vi "loop timing.vi"() -> ()   [LabVIEW 2013]
uses:
  <vilib>/DAQmx/read.llb/DAQmx Read (Digital Bool 1Line 1Point).vi
  <vilib>/DAQmx/write.llb/DAQmx Write (Digital Bool 1Line 1Point).vi
  <vilib>/DAQmx/create/channels.llb/DAQmx Create Channel (DI-Digital Input).vi
  <vilib>/DAQmx/create/channels.llb/DAQmx Create Channel (DO-Digital Output).vi
  <vilib>/DAQmx/miscellaneous.llb/DAQmx Fill In Error Info.vi
panel:
  out "error out 2":errorcluster
  out "error out":errorcluster
  in  "DAQmx DO":tag="Dev1/port0/line1"
  in  "DAQmx DI":tag="Dev1/port0/line0"
  out "Max":dbl=8.0 format="%_6g"
  in  "stop":bool
  out "Average":dbl=1.0015833898416784 format="%_6g"
  out "Delay":dbl=1.0 format="%_6g"
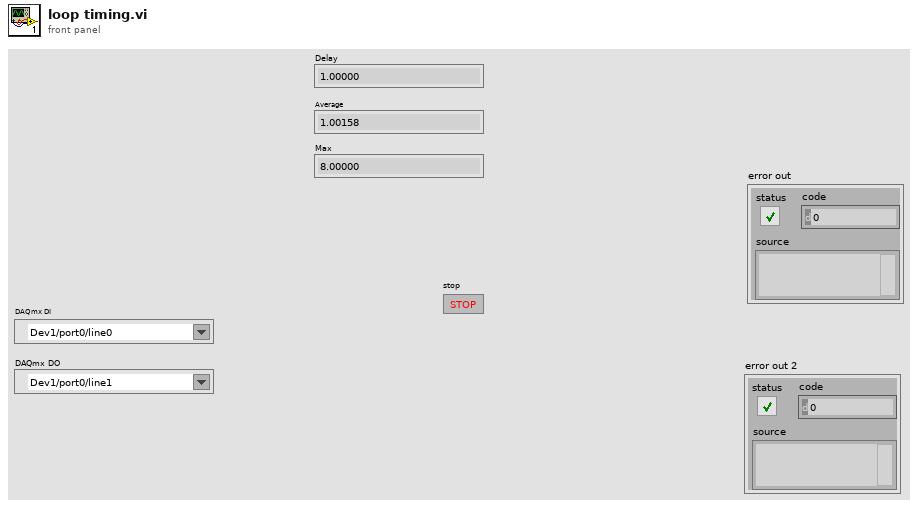
[diagram p1: front panel]
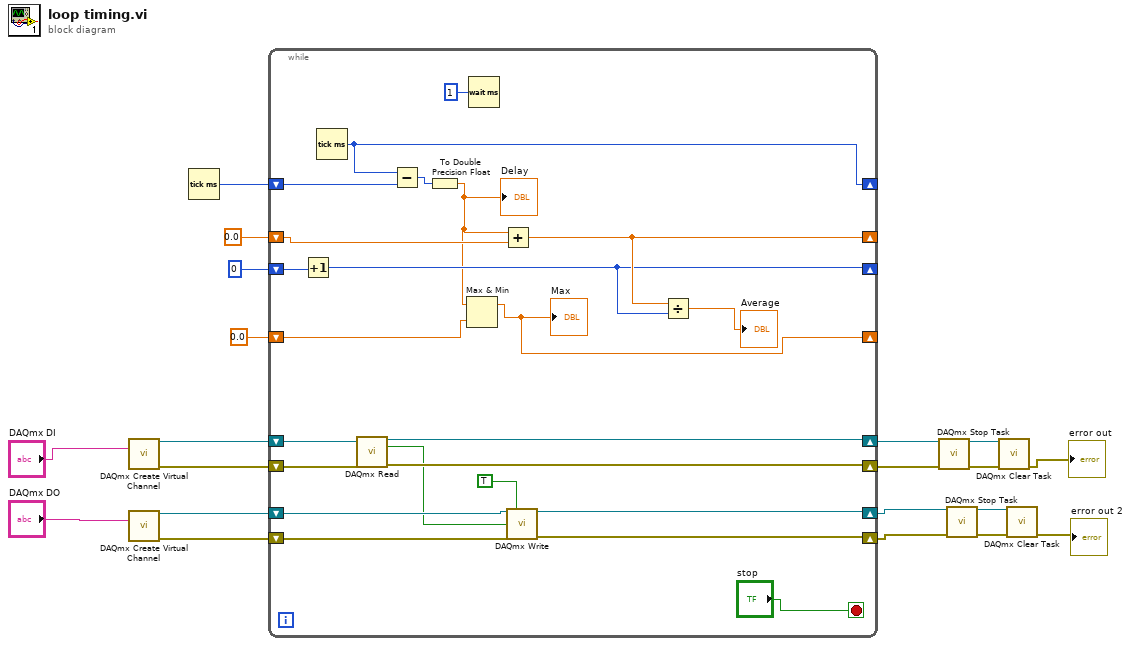
[diagram p0: block diagram]
diagram:
  n1 = call-poly <vilib>:"DAQmx Create Virtual Channel.vi"("lines"="DAQmx DI") -> ("task out"=w14:refnum<k21>, "error out"=w11:errorcluster)  [unwired: 13 in]
  n2 = call-poly <vilib>:"DAQmx Create Virtual Channel.vi"("lines"="DAQmx DO") -> ("task out"=w13:refnum<k21>, "error out"=w12:errorcluster)  [unwired: 13 in]
  n3 = Tick Count (ms)() -> (millisecond timer value=w20:u32)
  n4 = while {
    shift-right: [w40] -> _
    shift-left: w20 -> [w41]
    shift-right: [w36] -> _
    shift-left: 0.0 -> [w38]
    shift-right: [w35] -> _
    shift-left: 0 -> [w39]
    shift-right: [w31] -> _
    shift-left: 0.0 -> [w33]
    shift-right: [w29] -> w6
    shift-left: w13 -> [w30]
    shift-right: [w24] -> w4
    shift-left: w14 -> [w26]
    shift-right: [w27] -> w5
    shift-left: w12 -> [w28]
    shift-right: [w23] -> w3
    shift-left: w11 -> [w25]
    stop <- "stop" stop-if-true
    n5 = Increment(x=w39) -> (x+1=w35:i32)
    n6 = Tick Count (ms)() -> (millisecond timer value=w40:u32)
    n7 = call-poly <vilib>:"DAQmx Read.vi"("task/channels in"=w26, "error in"=w25) -> ("task out"=w24:refnum<k21>, "data"=w21:bool, "error out"=w23:errorcluster)  [unwired: 11 in]
    n8 = Subtract(x=w40, y=w41) -> (x-y=w37:u32)
    n9 = To Double Precision Float(number=w37) -> (double precision float=w32:dbl)
    "Delay" <- w32
    n10 = Max & Min(x=w32, y=w33) -> (max(x,y)=w31:dbl)  [unwired: 1 out]
    "Max" <- w31
    n11 = Wait (ms)(milliseconds to wait=u32 1) -> ()  [unwired: 1 out]
    n12 = Add(x=w32, y=w38) -> (x+y=w36:dbl)
    n13 = call-poly <vilib>:"DAQmx Write.vi"("task/channels in"=w30, "auto start"=TRUE, "data"=w21, "error in"=w28) -> ("task out"=w29:refnum<k21>, "error out"=w27:errorcluster)  [unwired: 9 in, 1 out]
    n14 = Divide(x=w36, y=w35) -> (x/y=→"Average":dbl)
  }
  n15 = call <vilib>:"DAQmx Stop Task.vi"("task/channels in"=w4, "error in"=w3) -> ("task out"=w10:refnum<k21>, "error out"=w9:errorcluster)  [unwired: 12 in]
  n16 = call <vilib>:"DAQmx Stop Task.vi"("task/channels in"=w6, "error in"=w5) -> ("task out"=w8:refnum<k21>, "error out"=w7:errorcluster)  [unwired: 12 in]
  n17 = call <vilib>:"DAQmx Clear Task.vi"("task in"=w10, "error in"=w9) -> ("error out"=→"error out":errorcluster)  [unwired: 13 in]
  n18 = call <vilib>:"DAQmx Clear Task.vi"("task in"=w8, "error in"=w7) -> ("error out"=→"error out 2":errorcluster)  [unwired: 13 in]
